vi "estimateDistanceToBreakBasedOnModel.vi"(8 "error in (no error)":errorcluster, 11 "Game in":refnum<class "Game.lvclass">) -> (0 "error out":errorcluster, 3 "Game out":refnum<class "Game.lvclass">)   [LabVIEW 2021, in "Game.lvclass"]
uses:
  Game.lvclass
  <vilib>/Analysis/baseanly.llb/Unit Vector (DBL).vi
  <vilib>/Analysis/baseanly.llb/A x Vector.vi
  <vilib>/Analysis/baseanly.llb/Real Dot Product.vi
  <vilib>/Analysis/NI_AALBase.lvlib
panel:
  in  "stateSpace":dbl[][](array[numeric])
  out "Waveform Chart":dbl[](graph)
  out "Boolean":bool
  in  "y":i32=2
  out "X * Y":dbl
  out "output array 2":dbl[][](array[numeric])
  out "output array":dbl[][](array[numeric])
  in  "target":dbl[](array[numeric])
  in  "v_sample":dbl=1.5
  in  "delta":dbl=0.1
  in  "position":dbl[](array[numeric])=[0.0, 0.0]
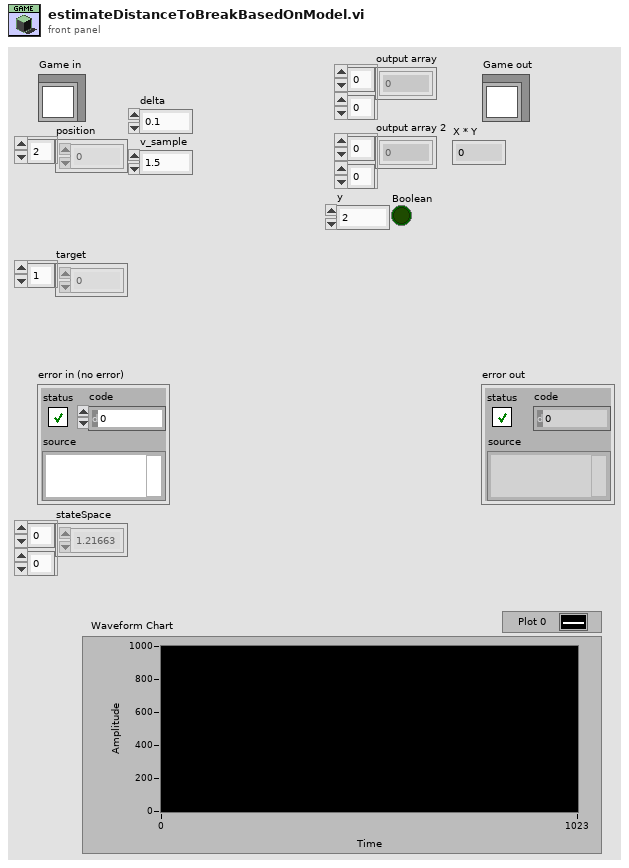
[diagram p1: front panel]
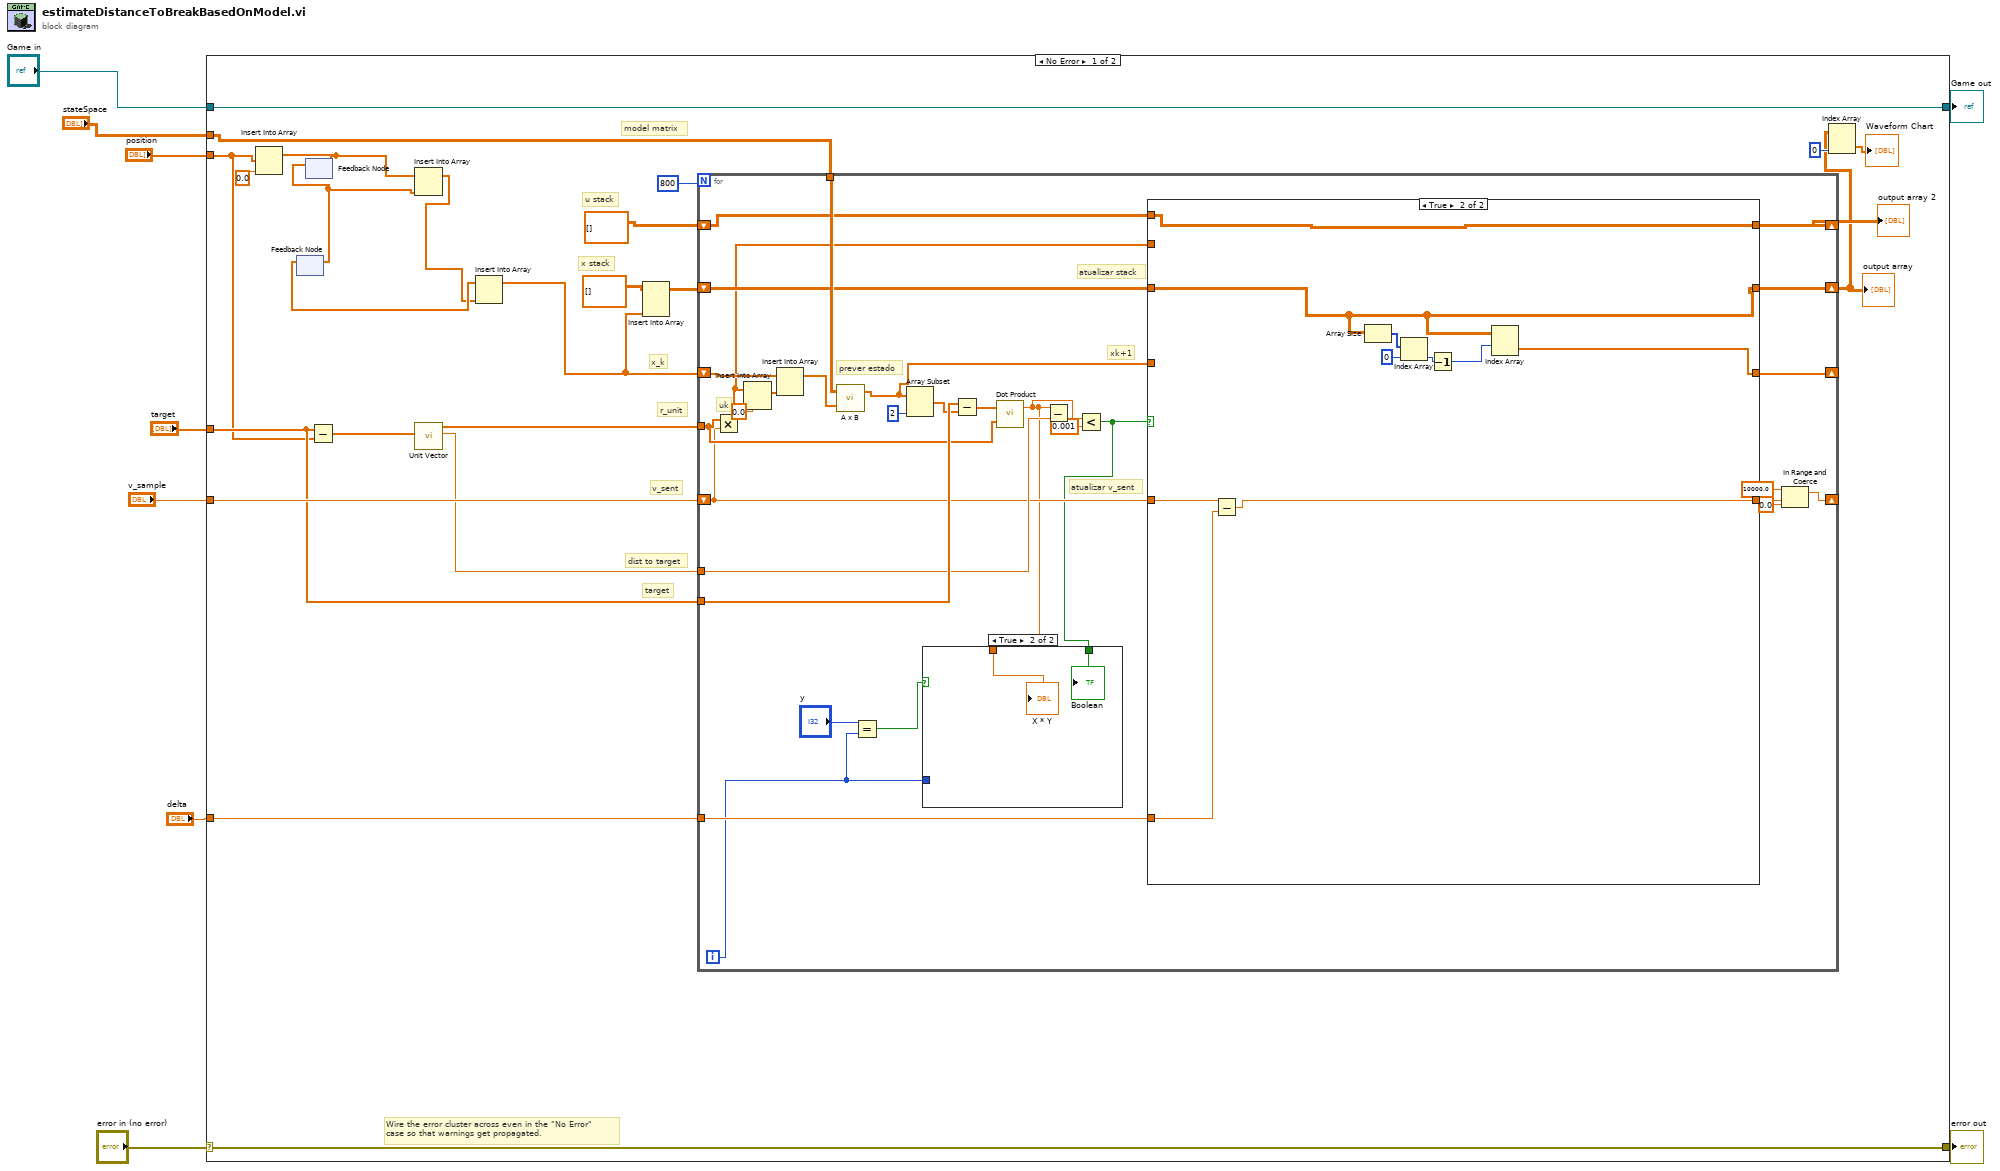
[diagram p0: block diagram]
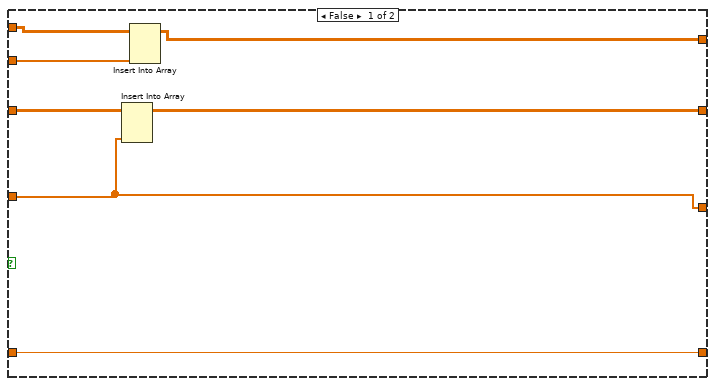
[diagram p3: hidden frame]
diagram:
  n1 = case shown="No Error" "error in (no error)" {
    selector: "error in (no error)" -> [w32 w84]
    tunnel: [w32 w84] -> w8
    tunnel: [w33 w83] -> w6
    tunnel: "Game in" -> [w33 w83]
    tunnel: "stateSpace" -> [w25 _]
    tunnel: "position" -> [w16 _]
    tunnel: "target" -> [w24 _]
    tunnel: "v_sample" -> [w26 _]
    tunnel: "delta" -> [w22 _]
    frame No Error {
      # "u stack"
      # "target"
      # "dist to target"
      # "model matrix"
      # "v_sent"
      # "r_unit"
      # "x_k"
      # "x stack"
      # "Wire the error cluster across even in the \"No Error\"\ncase so that warnings get propagated."
      n2 = Insert Into Array(array=w16, new element=0.0 ("new element/subarray")) -> (w15:dbl[])  [unwired: 1 in]
      n3 = feedback #1() -> (w30:dbl[])  [unwired: 1 in]
      n4 = feedback-in #2(w15) -> ()
      n5 = feedback #2() -> (w31:dbl[])  [unwired: 1 in]
      n6 = feedback-in #1(w31) -> ()
      n7 = Subtract(x=w24, y=w16) -> (x-y=w29:dbl[])
      n8 = Insert Into Array(array=w15, new element=w31) -> (w18:dbl[])  [unwired: 1 in]
      n9 = call-poly <vilib>:"Unit Vector.vi"("Input Vector"=w29) -> ("norm"=w23:dbl, "Unit Vector"=w27:dbl[])  [unwired: 8 in, 1 out]
      n10 = Insert Into Array(array=w30, new element=w18) -> (w20:dbl[])  [unwired: 1 in]
      n11 = Insert Into Array(array=dbl[][] [] ("output array"), new element=w20) -> (w19:dbl[][])  [unwired: 2 in]
      n12 = for {
        N: 800 -> [_]
        shift-right: [w53] -> w10
        shift-left: w19 -> [w54]
        shift-right: [w49] -> _
        shift-left: w20 -> [w50]
        tunnel: w27 -> [w57]
        shift-right: [w36] -> _
        shift-left: w26 -> [w52]
        tunnel: w25 -> [w63]
        tunnel: w24 -> [w60]
        tunnel: w23 -> [w56]
        tunnel: w22 -> [w51]
        shift-right: [w43] -> w13
        shift-left: dbl[][] [] ("output array") -> [w45]
        i -> [w42]
        # "xk+1"
        # "atualizar v_sent"
        # "atualizar stack"
        # "prever estado"
        # "uk"
        n13 = Multiply(x=w57, y=w52) -> (x*y=w44:dbl[])
        n14 = Insert Into Array(array=w44, new element=0.0 ("new element/subarray")) -> (w46:dbl[])  [unwired: 1 in]
        n15 = Insert Into Array(array=w50, new element=w46) -> (w62:dbl[])  [unwired: 1 in]
        n16 = call-poly <vilib>:"A x B.vi"("Vector"=w62, "A"=w63) -> ("A x Vector"=w48:dbl[])  [unwired: 1 out]
        n17 = Equal?(x="y", y=w42) -> (x = y?=w40:bool)
        n18 = Array Subset(array=w48, length=2) -> (w59:dbl[])  [unwired: 1 in]
        n19 = Subtract(x=w60, y=w59) -> (x-y=w58:dbl[])
        n20 = call-poly <vilib>:"Dot Product.vi"("Y Vector"=w57, "X Vector"=w58) -> ("X * Y"=w38:dbl)  [unwired: 1 out]
        n21 = Subtract(x=w38, y=w56) -> ()  [unwired: 1 out]
        n22 = Less?(x=w38, y=0.001) -> (x < y?=w39:bool)
        n23 = case shown="True" w40 {
          tunnel: w42 -> [_ _]
          tunnel: w38 -> [_ w65]
          tunnel: w39 -> [_ w64]
          frame False {
          }
          frame True {
            "X * Y" <- w65
            "Boolean" <- w64
          }
        }
        n24 = case shown="True" w39 {
          tunnel: w54 -> [w72 w77]
          tunnel: [w71 w77] -> w53
          tunnel: w52 -> [w70 w82]
          tunnel: w51 -> [_ w81]
          tunnel: [w70 w80] -> w37
          tunnel: [w69 w78] -> w49
          tunnel: w48 -> [w69 _]
          tunnel: w45 -> [w68 w79]
          tunnel: w44 -> [w67 _]
          tunnel: [w66 w79] -> w43
          frame False {
            n25 = Insert Into Array(array=w72, new element=w69) -> (w71:dbl[][])  [unwired: 2 in]
            n26 = Insert Into Array(array=w68, new element=w67) -> (w66:dbl[][])  [unwired: 2 in]
          }
          frame True {
            n27 = Subtract(x=w82, y=w81) -> (x-y=w80:dbl)
            n28 = Array Size(array=w77) -> (size(s)=w76:i32[])
            n29 = Index Array(array=w76, index=0) -> (element=w74:i32)
            n30 = Decrement(x=w74) -> (x-1=w73:i32)
            n31 = Index Array(array=w77, index (row)=w73) -> (element=w78:dbl[])  [unwired: 1 in]
          }
        }
        n32 = In Range and Coerce(upper limit=10000.0, x=w37, lower limit=0.0) -> (coerced(x)=w36:dbl)  [unwired: 1 out]
      }
      "output array" <- w10
      "output array 2" <- w13
      n33 = Index Array(array=w10, index (col)=0 ("disabled index (col)")) -> (element=→"Waveform Chart":dbl[])  [unwired: 1 in]
    }
    frame Error {
    }
  }
  "error out" <- w8
  "Game out" <- w6
